vi "Dashboard Main.vi"() -> ()   [LabVIEW 2017]
uses:
  <vilib>/Rock Robotics/Network Tables/NT Read Numeric Array.vi
  <vilib>/Rock Robotics/Network Tables/NT Read Number.vi
  <vilib>/Rock Robotics/Network Tables/NT Write Boolean.vi
  <vilib>/Rock Robotics/Network Tables/NT Write Number.vi
panel:
  out "Camera Info":cluster{"Mbps LED":bool, "Mbps":dbl, "fps":dbl} {"fps" format="%#.1g"; "Mbps" format="%#.1g"}
  in  "Camera Settings":T1={"Frame Rate"=30, "Compression"=30, "Size"=1, "DB Camera Config"=FALSE} {"Frame Rate" scale=1.0..30.0; "Compression" scale=100.0..-1.0; "Size" items=["640x480", "320x240", "160x120"]}
  in  "TCP":refnum<k5>
  out "Robot IP":string
  in  "Dashboard Tab":enum32{"Drive", "Basic", "Custom", "Variables"}(tab)
  out "Accel mins":dbl[](array[numeric])
  in  "Boolean":bool
  out "AvgY":dbl
  out "AvgX":dbl
  out "Accel maxs":dbl[](array[numeric])
  out "Accels":dbl[](array[numeric])
  out "Gyro rate":dbl
  out "Gyro":dbl
  in  "Select Auto":string(combo)="Select Autonomous ..."
  out "NT Connection":bool
  out "MotorChart R":cluster{"Numeric":dbl, "Numeric":dbl}(graph)
  out "MotorChart L":cluster{"Numeric":dbl, "Numeric":dbl}(graph)
  out "MotorSliders R":cluster{"MotorSlide1":dbl, "MotorSlide2":dbl} {"MotorSlide2" scale=-1.0..1.0 scale format="%#_2e"; "MotorSlide1" scale=-1.0..1.0 scale format="%#_2e"}
  out "MotorSliders L":cluster{"MotorSlide1":dbl, "MotorSlide2":dbl} {"MotorSlide2" scale=-1.0..1.0 scale format="%#_2e"; "MotorSlide1" scale=-1.0..1.0 scale format="%#_2e"}
  out "JS1 Z":dbl(slide) scale=-1.0..1.0 scale format="%#_2e"
  out "JS1 Graph":cluster{"X":dbl, "Y":dbl}[](graph)
  out "JS1 Buttons":T2
  out "JS2 Z":dbl(slide) scale=-1.0..1.0 scale format="%#_2e"
  out "JS2 Graph":cluster{"X":dbl, "Y":dbl}[](graph)
  out "JS2 Buttons":T2
  out "Mode":T3(ring)=enum."Auto Disabled"
  in  "DB/String 9":string
  in  "DB/String 8":string
  in  "DB/String 7":string
  in  "DB/String 6":string
  in  "DB/String 5":string
  in  "DB/String 4":string
  in  "DB/String 3":string
  in  "DB/String 2":string
  in  "DB/String 1":string
  in  "DB/String 0":string
  in  "DB/Slider 0":dbl(slide) scale=0.0..5.0
  in  "DB/Slider 1":dbl(slide) scale=0.0..5.0
  in  "DB/Slider 2":dbl(slide) scale=0.0..5.0
  in  "DB/Slider 3":dbl(slide) scale=0.0..5.0
  out "DB/LED 3":bool
  out "DB/LED 2":bool
  out "DB/LED 1":bool
  out "DB/LED 0":bool
  in  "DB/Button 3":bool
  in  "DB/Button 2":bool
  in  "DB/Button 1":bool
  in  "DB/Button 0":bool caption="New Name"
  in  "x":dbl
  in  "y":dbl
  in  "y off":dbl
  in  "x off":dbl
  out "Tree":string(tree)
  out "Camera Image":T4(plugin-control)
  out "Background":bool
  in  "Camera Name":string(combo)="No Camera Selection"
  # "HW"
  # "Joysticks"
  # "Drive Motors"
  # "Front"
  # "Right"
  # "Left"
  # "Back"
  # "This tab is a great place for autonomous settings and robot-specific values.\nPlace controls and indicators inside this tab and match name to\nDashboard Variables on robot. You can also delete this comment."
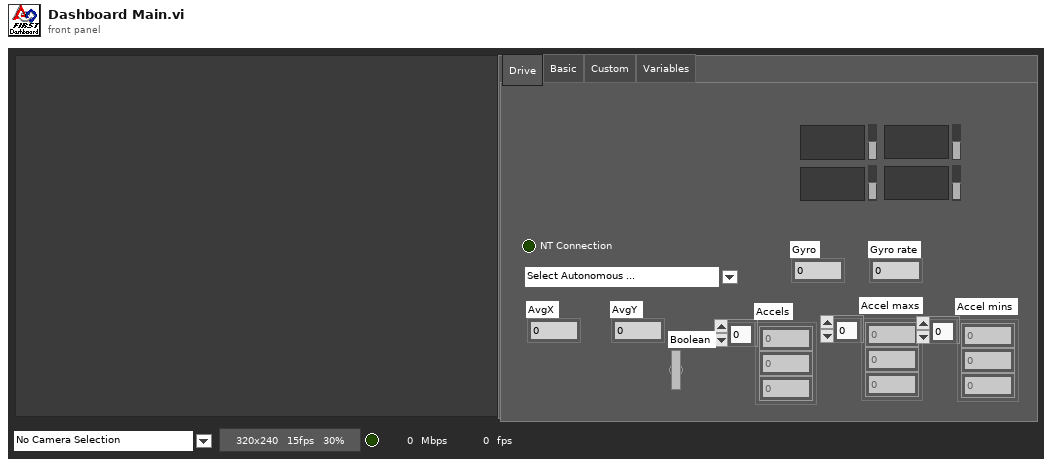
[diagram p1: front panel]
types:
  T1 = cluster{"Frame Rate":i32, "Compression":i32, "Size":u16, "DB Camera Config":bool}
  T2 = cluster{bool, bool, bool, bool, bool, bool, bool, bool, bool, bool, bool, bool}
  T3 = enum8{"Tele-Op Disabled", "Tele-Op Enabled", "Auto Disabled", "Auto Enabled", "Test Disabled", "Test Enabled", "Disconnected", "No Code", "E-Stop"}
  T4 = typedef "IMAQ Image.ctl" = refnum<image>
  T5 = cluster{"Save Path":path, "Interval (s)":dbl, "Keep":i32}
  T6 = typedef "Image Type" = u32
  T7 = cluster{"Camera Image":refnum<vi>, "Dashboard Tab":refnum<vi>, "Background":refnum<vi>, "Tree":refnum<vi>, "Camera Settings":refnum<vi>, "Camera Name":refnum<vi>, "Camera Info":refnum<vi>}
  T8 = cluster{"Error Strings":string, "Disable Counts":cluster{u16, u16}, "Rail Faults":cluster{u16, u16, u16}, "Robot IP":string, "DB Mode":u8, "Event Info":cluster{"Name":string, "Type":u8, "Number":u16, "Replay":u8}}
  T9 = cluster{"Storage":cluster{"Disk Free":u64, "RAM Block":u32, "RAM free":u32}, "CPU Utilization":cluster{"CPU % ISR":sgl, "CPU % Time Crit":sgl, "CPU % Timed Str":sgl, "CPU % High":sgl, "CPU % Above":sgl, "CPU % Normal":sgl, "CPU % Low":sgl}, "CAN":cluster{"% Bus Utilization":sgl, "Bus Off Cnt":u32, "TX_FIFO Full Cnt":u32, "Receive Error Cnt":u8, "Transmit Error Cnt":u8}, "HID":cluster{"HID Outputs":u32, "Rumble Low":u16, "Rumble High":u16}[]}
  T10 = cluster{"Status bits":cluster{"Test Mode":bool, "Autonomous":bool, "Enabled":bool, "Code Start":bool, "Brownout":bool, "Reserved 2":bool, "Reserved 3":bool, "E-Stop":bool}, "Code Trace":cluster{"Disabled":bool, "TeleOp":bool, "Auto":bool, "Test":bool}, "Controller Type":enum16{"unknown", "cRIO", "roboRio"}, "Code?":enum16{"unknown", "noCode", "code"}, "Battery V":dbl}
  T11 = cluster{"Control Bits":cluster{"TestMode":bool, "Autonomous":bool, "Enabled":bool, "FMS Present":bool, bool, bool, bool, "E-Stop":bool}, "Team Station ":u8, "Countdown":sgl, "Joystick Values":cluster{"Axes":dbl[], "Buttons":bool[], "POVs":i16[]}[]}
  T12 = cluster{"Axes":dbl[], "Buttons":bool[], "POVs":i16[]}[]
  T13 = cluster{"Axes":dbl[], "Buttons":bool[], "POVs":i16[]}
  T14 = cluster{"Buttons[0]":bool, "Buttons[1]":bool, "Buttons[2]":bool, "Buttons[3]":bool, "Buttons[4]":bool, "Buttons[5]":bool, "Buttons[6]":bool, "Buttons[7]":bool, "Buttons[8]":bool, "Buttons[9]":bool, "Buttons[10]":bool, "Buttons[11]":bool}
  T15 = cluster{"Shift":bool, "Ctrl":bool, "Alt":bool, "Cmd":bool, "Opt":bool}
  T16 = cluster{"Camera Name":string, "Camera File Name":string, "Saved DB Images Info":cluster{"Save Path":path, "Interval (s)":dbl, "Keep":i32}}
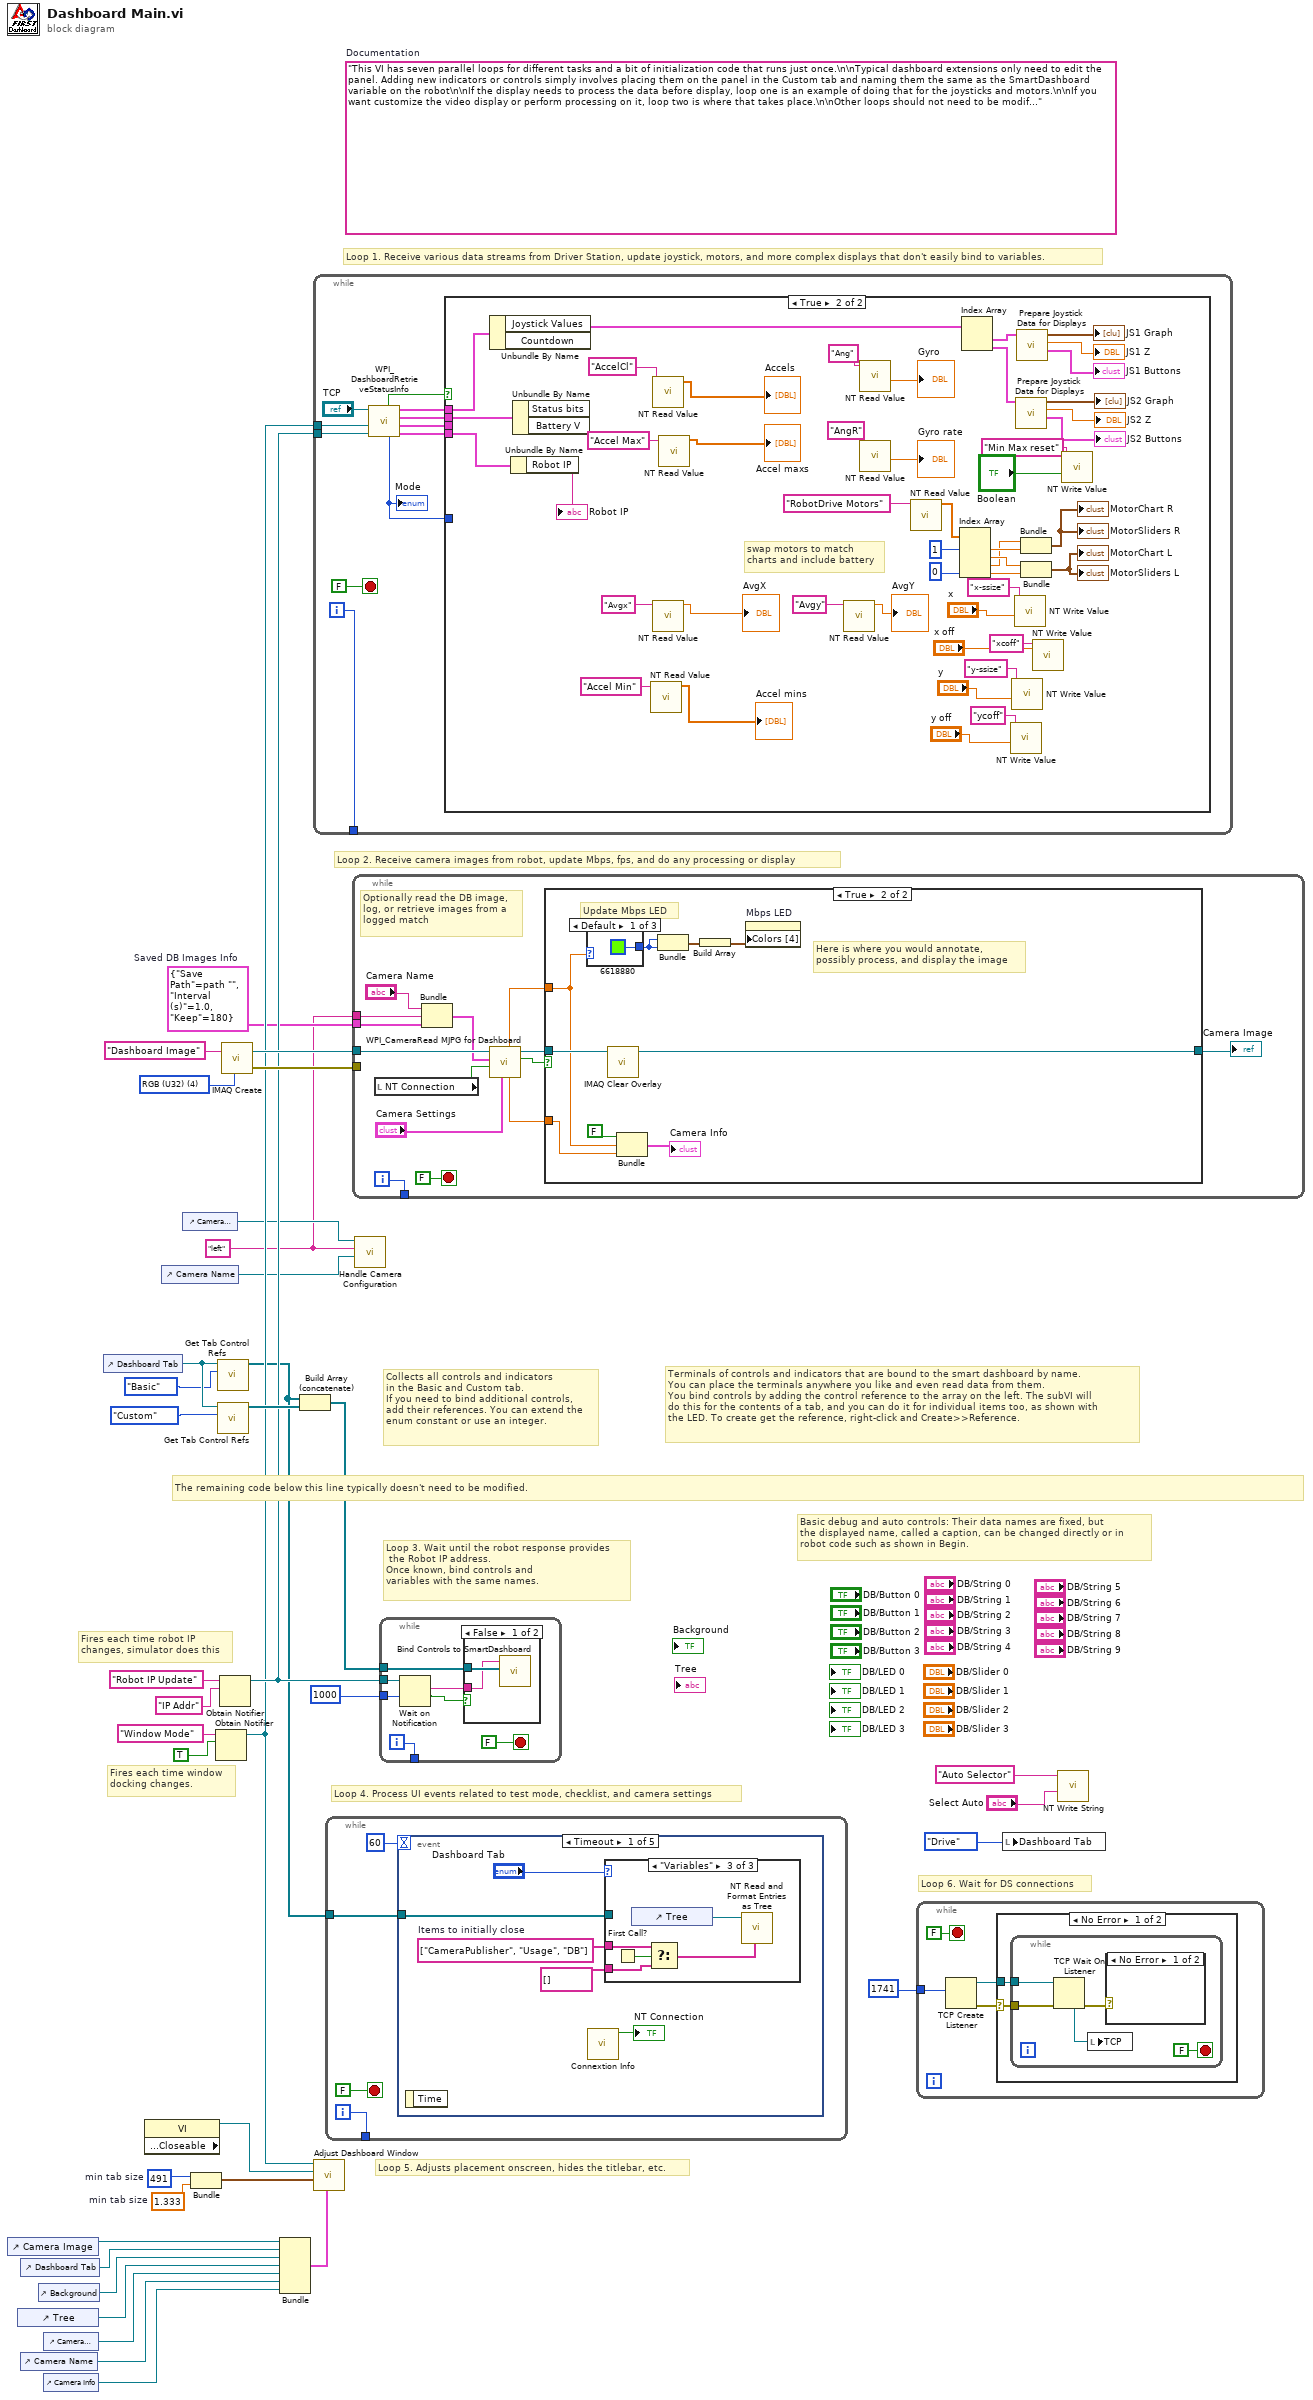
[diagram p0: block diagram]
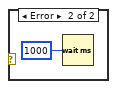
[diagram p2: hidden frame]
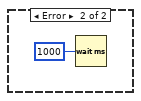
[diagram p3: hidden frame]
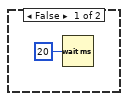
[diagram p4: hidden frame]
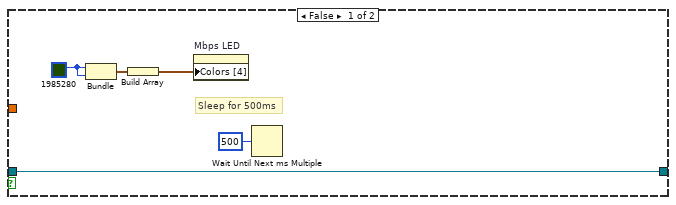
[diagram p6: hidden frame]
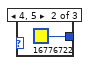
[diagram p7: hidden frame]
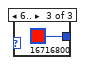
[diagram p8: hidden frame]
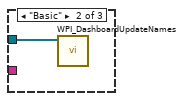
[diagram p10: hidden frame]
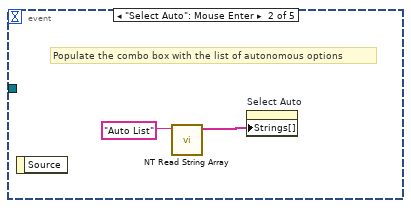
[diagram p11: hidden frame]
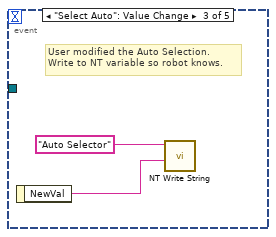
[diagram p12: hidden frame]
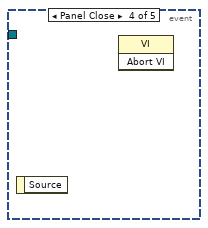
[diagram p13: hidden frame]
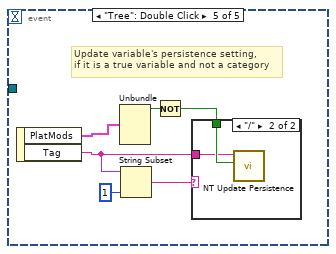
[diagram p14: hidden frame]
diagram:
  w1 = "left" ("Camera File Name")
  w2 = T5 {"Save Path"=path "", "Interval (s)"=1.0, "Keep"=180}  # Saved DB Images Info
  w22 = 491  # min tab size
  w21 = 1.333  # min tab size
  (unwired) "This VI has seven parallel loops for different tasks and a bit of initialization code that runs just once.\n\nTypical dashboard extensions only need to edit the panel. Adding new indicators or controls simply involves placing them on the panel in the Custom tab and naming them the same as the SmartDashboard variable on the robot\n\nIf the display needs to process the data before display, loop one is an example of doing that for the joysticks and motors.\n\nIf you want customize the video display or perform processing on it, loop two is where that takes place.\n\nOther loops should not need to be modified. They are pretty standard, and document the task they perform."  # Documentation
  w37 = T6 4 items=["Grayscale (U8)", "Grayscale (I16)", "Grayscale (SGL)", "Complex (CSG)", "RGB (U32)", "HSL (U32)", "RGB (U64)"] ("Image Type")
  # "Loop 6. Wait for DS connections"
  # "Basic debug and auto controls: Their data names are fixed, but\nthe displayed name, called a caption, can be changed directly or in\nrobot code such as shown in Begin."
  # "Fires each time robot IP\nchanges, simulator does this"
  # "Fires each time window\ndocking changes."
  # "Collects all controls and indicators\nin the Basic and Custom tab.\nIf you need to bind additional controls,\nadd their references. You can extend the\nenum constant or use an integer."
  # "The remaining code below this line typically doesn't need to be modified."
  # "Loop 4. Process UI events related to test mode, checklist, and camera settings"
  # "Terminals of controls and indicators that are bound to the smart dashboard by name.\nYou can place the terminals anywhere you like and even read data from them.\nYou bind controls by adding the control reference to the array on the left. The subVI will\ndo this for the contents of a tab, and you can do it for individual items too, as shown with\nthe LED. To create get the reference, right-click and Create>>Reference."
  # "Loop 3. Wait until the robot response provides\n the Robot IP address.\nOnce known, bind controls and\nvariables with the same names."
  # "Loop 5. Adjusts placement onscreen, hides the titlebar, etc."
  # "Loop 1. Receive various data streams from Driver Station, update joystick, motors, and more complex displays that don't easily bind to variables."
  # "Loop 2. Receive camera images from robot, update Mbps, fps, and do any processing or display"
  n1 = control-ref of="Camera Image"() -> (w24:refnum<vi>)
  n2 = control-ref of="Tree"() -> (w8:refnum<vi>)
  n3 = control-ref of="Dashboard Tab"() -> (w23:refnum<vi>)
  n4 = control-ref of="Camera Name"() -> (w6:refnum<vi>)
  n5 = control-ref of="Background"() -> (w19:refnum<vi>)
  n6 = control-ref of="Camera Settings"() -> (w7:refnum<vi>)
  n7 = control-ref of="Camera Info"() -> (w5:refnum<vi>)
  n8 = control-ref of="Dashboard Tab"() -> (w27:refnum<vi>)
  n9 = property class="VI" props=["Front Panel.Closeable"]() -> (reference out=w28:refnum<vi>)  [unwired: 2 in, 2 out]
  n10 = control-ref of="Camera Name"() -> (w12:refnum<vi>)
  n11 = control-ref of="Camera Settings"() -> (w13:refnum<vi>)
  n12 = Bundle("min tab size"=w22, "min tab size"=w21) -> (w20:cluster{"min tab size":i32, "min tab size":dbl})  [unwired: 1 in]
  n13 = Obtain Notifier(name (unnamed)="Window Mode", notification data type=TRUE) -> (notifier out=w16:refnum<notifier>)  [unwired: 2 in, 2 out]
  n14 = call <vilib>:"Get Tab Control Refs.vi"("Page Index"=enum32{"Drive", "Basic", "Custom", "Variables"}."Basic" ("Dashboard Tab"), "TabControl in"=w27) -> ("ControlsOnPage"=w11:refnum<vi>[])  [unwired: 9 in]
  n15 = call <vilib>:"Get Tab Control Refs.vi"("Page Index"=enum32{"Drive", "Basic", "Custom", "Variables"}."Custom" ("Dashboard Tab"), "TabControl in"=w27) -> ("ControlsOnPage"=w26:refnum<vi>[])  [unwired: 9 in]
  n16 = Obtain Notifier(name (unnamed)="Robot IP Update", notification data type="IP Addr" ("name (unnamed)")) -> (notifier out=w17:refnum<notifier>)  [unwired: 2 in, 2 out]
  n17 = call "IMAQ Create"("Image Name"="Dashboard Image", "Image Type"=w37) -> ("New Image"=w35:T4, "error out"=w34:errorcluster)  [unwired: 2 in, 1 out]
  n18 = Bundle("Camera Image"=w24, "Dashboard Tab"=w23, "Background"=w19, "Tree"=w8, "Camera Settings"=w7, "Camera Name"=w6, "Camera Info"=w5) -> (w18:T7)  [unwired: 1 in]
  n19 = Build Array (concatenate)(w11, w26) -> (w25:refnum<vi>[])
  n20 = while {
    tunnel: [w47] -> _
    tunnel: w17 -> [w41]
    tunnel: w16 -> [w38]
    i -> [w47]
    stop <- FALSE stop-if-true
    n21 = call <vilib>:"WPI_DashboardRetrieveStatusInfo.vi"("Binding Refnum"=w41, "Window Mode Notifier"=w38, "TCP Cnx"="TCP") -> ("Power and Errors"=w42:T8, "Robot Metrics"=w45:T9, "Status Info"=w46:T10, "Control Info"=w43:T11, "Robot Mode"=w40:T3, "Process?"=w44:bool)  [unwired: 3 in]
    "Mode" <- w40
    n22 = case shown="True" w44 {
      tunnel: w46 -> [_ w96]
      tunnel: w45 -> [_ _]
      tunnel: w43 -> [_ w95]
      tunnel: w42 -> [_ w94]
      tunnel: w40 -> [_ _]
      frame False {
        n23 = Wait (ms)(milliseconds to wait=u32 20) -> ()  [unwired: 1 out]
      }
      frame True {
        # "swap motors to match\ncharts and include battery"
        n24 = Unbundle By Name(w95) -> ("Joystick Values"=w85:T12)  [unwired: 1 out]
        n25 = Unbundle By Name(w94) -> ("Robot IP"=→"Robot IP":string)
        n26 = Unbundle By Name(w96) -> ()  [unwired: 2 out]
        n27 = call-poly <vilib>:"NT Read Value.vi"("Name"="Accel Min") -> ("Numeric Array"=→"Accel mins":dbl[])  [unwired: 9 in, 1 out]
        n28 = call-poly <vilib>:"NT Read Value.vi"("Name"="AccelCl") -> ("Numeric Array"=→"Accels":dbl[])  [unwired: 9 in, 1 out]
        n29 = call-poly <vilib>:"NT Read Value.vi"("Name"="Avgx") -> ("Numeric"=→"AvgX":dbl)  [unwired: 9 in, 1 out]
        n30 = call-poly <vilib>:"NT Read Value.vi"("Name"="Accel Max") -> ("Numeric Array"=→"Accel maxs":dbl[])  [unwired: 9 in, 1 out]
        n31 = call-poly <vilib>:"NT Read Value.vi"("Name"="Avgy") -> ("Numeric"=→"AvgY":dbl)  [unwired: 9 in, 1 out]
        n32 = call-poly <vilib>:"NT Read Value.vi"("Name"="Ang") -> ("Numeric"=→"Gyro":dbl)  [unwired: 9 in, 1 out]
        n33 = call-poly <vilib>:"NT Read Value.vi"("Name"="AngR") -> ("Numeric"=→"Gyro rate":dbl)  [unwired: 9 in, 1 out]
        n34 = call-poly <vilib>:"NT Read Value.vi"("Name"="RobotDrive Motors") -> ("Numeric Array"=w75:dbl[])  [unwired: 9 in, 1 out]
        n35 = Index Array(array=w75, index #1=1, index #4=0) -> (element #1=w89:dbl, element #2=w90:dbl, element #3=w88:dbl, element #4=w93:dbl)  [unwired: 2 in]
        n36 = Index Array(array=w85) -> (element #1=w84:T13, element #2=w80:T13)  [unwired: 2 in]
        n37 = call-poly <vilib>:"NT Write Value.vi"("Numeric"="y off", "Name"="ycoff") -> ()  [unwired: 9 in, 1 out]
        n38 = call-poly <vilib>:"NT Write Value.vi"("Numeric"="y", "Name"="y-ssize") -> ()  [unwired: 9 in, 1 out]
        n39 = call-poly <vilib>:"NT Write Value.vi"("Numeric"="x", "Name"="x-ssize") -> ()  [unwired: 9 in, 1 out]
        n40 = call "Prepare Joystick Data for Displays.vi"("Joystick Values"=w80) -> ("Buttons"=→"JS2 Buttons":T14, "Z Axis"=→"JS2 Z":dbl, "Cartesian Data"=→"JS2 Graph":cluster{"X axis":dbl, "X axis":dbl}[])  [unwired: 8 in]
        n41 = call "Prepare Joystick Data for Displays.vi"("Joystick Values"=w84) -> ("Buttons"=→"JS1 Buttons":T14, "Z Axis"=→"JS1 Z":dbl, "Cartesian Data"=→"JS1 Graph":cluster{"X axis":dbl, "X axis":dbl}[])  [unwired: 8 in]
        n42 = Bundle("Numeric"=w88, "Numeric"=w89) -> (→"MotorChart R" →"MotorSliders R":cluster{"Numeric":dbl, "Numeric":dbl})  [unwired: 1 in]
        n43 = Bundle("Numeric"=w90, "Numeric"=w93) -> (→"MotorChart L" →"MotorSliders L":cluster{"Numeric":dbl, "Numeric":dbl})  [unwired: 1 in]
        n44 = call-poly <vilib>:"NT Write Value.vi"("Numeric"="x off", "Name"="xcoff") -> ()  [unwired: 9 in, 1 out]
        n45 = call-poly <vilib>:"NT Write Value.vi"("Boolean"="Boolean", "Name"="Min Max reset") -> ()  [unwired: 9 in, 1 out]
      }
    }
  }
  n46 = call "Adjust Dashboard Window.vi"("Sizing Refnums"=w18, "Size Constraints"=w20, "VI"=w28, "WIn Mode"=w16) -> ()  [unwired: 8 in]
  n47 = while {
    tunnel: [w98] -> _
    tunnel: w11 -> [w97]
    i -> [w98]
    stop <- FALSE stop-if-true
    n48 = event shown="[0] Timeout" {
      selector: _ -> [_ _ _ _ _]
      dyn-events: _ -> [_ _ _ _ _]
      timeout: u32 60 ("milliseconds to wait") -> [_ _ _ _ _]
      tunnel: w97 -> [w103 _ _ _ _]
      event Timeout {
        w102 = string[] ["CameraPublisher", "Usage", "DB"]  # Items to initially close
        n49 = event-data() -> ()  [unwired: 1 in, 1 out]
        n50 = call <vilib>:"Connextion Info.vi"() -> ("Connected"=→"NT Connection":bool)  [unwired: 10 in, 1 out]
        n51 = case shown="\"Variables\"" "Dashboard Tab" {
          tunnel: w103 -> [_ w106 _]
          tunnel: w102 -> [_ _ w109]
          tunnel: string[] [] -> [_ _ w108]
          frame "Custom", Default {
          }
          frame "Basic" {
            n52 = call <vilib>:"WPI_DashboardUpdateNames.vi"("Controls on Tab"=w106) -> ()  [unwired: 11 in]
          }
          frame "Variables" {
            n53 = First Call?() -> (First Call?: T/F=w110:bool)
            n54 = control-ref of="Tree"() -> (w111:refnum<vi>)
            n55 = Select(t=w109, s=w110, f=w108) -> (s? t:f=w107:string[])
            n56 = call <vilib>:"NT Read and Format Entries as Tree.vi"("Tags to  Close"=w107, "Tree Refnum"=w111) -> ()  [unwired: 8 in, 2 out]
          }
        }
      }
      event "Select Auto": Mouse Enter {
        # "Populate the combo box with the list of autonomous options"
        n57 = event-data() -> ()  [unwired: 1 in, 1 out]
        n58 = call <vilib>:"NT Read String Array.vi"("Name"="Auto List") -> ("String Array"=w112:string[])  [unwired: 9 in, 1 out]
        n59 = property on="Select Auto" class="CmbBox"("Strings[]"=w112) -> ()  [unwired: 2 in, 2 out]
      }
      event "Select Auto": Value Change {
        # "User modified the Auto Selection.\nWrite to NT variable so robot knows."
        n60 = event-data() -> ("NewVal"=w114:string)  [unwired: 1 in]
        n61 = call <vilib>:"NT Write String.vi"("String"=w114, "Name"="Auto Selector") -> ()  [unwired: 9 in, 1 out]
      }
      event Panel Close {
        n62 = event-data() -> ()  [unwired: 1 in, 1 out]
        n63 = invoke class="VI" method="Abort VI"() -> ()  [unwired: 3 in, 3 out]
      }
      event "Tree": Double Click {
        # "Update variable's persistence setting,\nif it is a true variable and not a category"
        n64 = event-data() -> ("PlatMods"=w117:T15, "Tag"=w116:string)  [unwired: 1 in]
        n65 = Unbundle(w117) -> ("Shift"=w121:bool)  [unwired: 4 out]
        n66 = String Subset(string=w116, length (rest)=1 ("length (rest)")) -> (substring=w118:string)  [unwired: 1 in]
        n67 = Not(x=w121) -> (.not. x?=w120:bool)
        n68 = case shown="\"/\"" w118 {
          tunnel: w120 -> [_ w123]
          tunnel: w116 -> [_ w122]
          frame Default {
          }
          frame "/" {
            n69 = call <vilib>:"NT Update Persistence.vi"("Persistence"=w123, "Name"=w122) -> ()  [unwired: 9 in, 1 out]
          }
        }
      }
    }
  }
  n70 = while {
    tunnel: w35 -> [w135]
    tunnel: w34 -> [_]
    tunnel: [w136] -> _
    tunnel: w2 -> [w127]
    tunnel: w1 -> [w124]
    i -> [w136]
    stop <- FALSE stop-if-true
    # "Optionally read the DB image,\nlog, or retrieve images from a\nlogged match"
    n71 = local read "NT Connection"() -> (w128:bool)
    n72 = Bundle("Camera Name"="Camera Name", "Camera File Name"=w124, "Saved DB Images Info"=w127) -> (w126:T16)  [unwired: 1 in]
    n73 = call <vilib>:"WPI_CameraRead MJPG for Dashboard.vi"("Camera Settings"="Camera Settings", "NT Connection"=w128, "Capture Info"=w126, "Refnum in"=w135) -> ("Active"=w133:bool, "Refnum out"=w134:T4, "FPS"=w132:dbl, "Bandwidth (Mbps)"=w131:dbl)  [unwired: 4 in]
    n74 = case shown="True" w133 {
      tunnel: w134 -> [w138 w149]
      tunnel: w131 -> [_ w146]
      tunnel: w132 -> [_ w147]
      tunnel: [w138 w143] -> w129
      frame False {
        w140 = u32 1985280 ("Color Box")
        # "Sleep for 500ms"
        n75 = Bundle("Color Box"=w140, "Color Box"=w140) -> (w141:cluster{"Color Box":u32, "Color Box":u32})  [unwired: 1 out]
        n76 = Build Array(w141) -> (w139:cluster{"Color Box":u32, "Color Box":u32}[])
        n77 = property on="Mbps LED" class="Bool (strict)"("Colors [4]"=w139) -> ()  [unwired: 2 in, 2 out]
        n78 = Wait Until Next ms Multiple(millisecond multiple=u32 500) -> ()  [unwired: 1 out]
      }
      frame True {
        # "Here is where you would annotate,\npossibly process, and display the image"
        # "Update Mbps LED"
        n79 = case shown="Default" w146 {
          tunnel: [u32 6618880 ("Color Box") u32 16776722 ("Color Box") u32 16716800 ("Color Box")] -> w150
          frame Default {
          }
          frame 4, 5 {
          }
          frame 6.. {
          }
        }
        n80 = call "IMAQ Clear Overlay"("Image"=w149) -> ("Image Out"=w143:T4)  [unwired: 2 in, 8 out]
        n81 = Bundle(FALSE, "Bandwidth (Mbps)"=w146, "FPS"=w147) -> (→"Camera Info":cluster{bool, "Bandwidth (Mbps)":dbl, "FPS":dbl})  [unwired: 1 in]
        n82 = Bundle("Color Box"=w150, "Color Box"=w150) -> (w151:cluster{"Color Box":u32, "Color Box":u32})  [unwired: 1 out]
        n83 = Build Array(w151) -> (w148:cluster{"Color Box":u32, "Color Box":u32}[])
        n84 = property on="Mbps LED" class="Bool (strict)"("Colors [4]"=w148) -> ()  [unwired: 2 in, 2 out]
      }
    }
    "Camera Image" <- w129
  }
  n85 = call "Handle Camera Configuration.vi"("CameraNameRef"=w12, "Camera File Name"=w1, "ClusterRef"=w13) -> ()  [unwired: 9 in]
  n86 = while {
    tunnel: w25 -> [w161]
    tunnel: w17 -> [w159]
    tunnel: [w157] -> _
    tunnel: u32 1000 ("milliseconds to wait") -> [w156]
    i -> [w157]
    stop <- FALSE stop-if-true
    n87 = Wait on Notification(notifier=w159, timeout in ms (-1)=w156) -> (notification=w158:string, timed out?=w155:bool)  [unwired: 2 in, 2 out]
    n88 = case shown="False" w155 {
      tunnel: w161 -> [w163 _]
      tunnel: w158 -> [w162 _]
      frame False {
        n89 = call <vilib>:"Bind Controls to SmartDashboard.vi"("Bound Control Refs"=w163, "Server IP Address"=w162) -> ()  [unwired: 10 in]
      }
      frame True {
      }
    }
  }
  n90 = while {
    tunnel: u16 1741 ("timeout ms (25000)") -> [w165]
    stop <- FALSE stop-if-true
    n91 = TCP Create Listener(10:w165) -> (0:w164:errorcluster, 3:w166:refnum<k5>)  [unwired: 4 in, 1 out]
    n92 = case shown="No Error" w164 {
      selector: w164 -> [w168 _]
      tunnel: w166 -> [w169 _]
      frame No Error {
        n93 = while {
          tunnel: w169 -> [w172]
          tunnel: w168 -> [w171]
          stop <- FALSE stop-if-true
          n94 = TCP Wait On Listener(8:w171, 11:w172) -> (0:w173:errorcluster, 4:w174:refnum<k5>)  [unwired: 2 in, 3 out]
          n95 = local write "TCP"(w174) -> ()
          n96 = case shown="No Error" w173 {
            frame No Error {
            }
            frame Error {
              n97 = Wait (ms)(milliseconds to wait=u32 1000) -> ()  [unwired: 1 out]
            }
          }
        }
      }
      frame Error {
        n98 = Wait (ms)(milliseconds to wait=u32 1000) -> ()  [unwired: 1 out]
      }
    }
  }
  n99 = local write "Dashboard Tab"(enum32{"Drive", "Basic", "Custom", "Variables"}."Drive" ("Dashboard Tab")) -> ()
  n100 = call <vilib>:"NT Write String.vi"("String"="Select Auto", "Name"="Auto Selector") -> ()  [unwired: 9 in, 1 out]
